vi "FindHome_SingleAxis.vi"(0 "Bd ID In":T3=1, 1 "Home Voltage":dbl, 5 "Axis":T1=1 items=["Axis 1"=1, "Axis 2"=2, "Axis 3"=3, "Axis 4"=4, "Axis 5"=5, "Axis 6"=6, "Axis 7"=7, "Axis 8"=8], 11 "error in":errorcluster, 12 "Velocity (RPM)":i32=65, 13 "Acceleration (RPS/s)":dbl=4.0 format="%.2f") -> (4 "Bd ID Out":T3, 6 "Axis Resource Output":T2 items=["Axis Control"=0, "Axis 1"=1, "Axis 2"=2, "Axis 3"=3, "Axis 4"=4, "Axis 5"=5, "Axis 6"=6, "Axis 7"=7, "Axis 8"=8, "Vector Space Control"=16, "Vector Space 1"=17, "Vector Space 2"=18, "Vector Space 3"=19, "Vector Space 4"=20, "Encoder Control"=32, "Encoder 1"=33, "Encoder 2"=34, "Encoder 3"=35, "Encoder 4"=36, "Encoder 5"=37, "Encoder 6"=38, "Encoder 7"=39, "Encoder 8"=40, "DAC Channel 1"=49, "DAC Channel 2"=50, "DAC Channel 3"=51, "DAC Channel 4"=52, "DAC Channel 5"=53, "DAC Channel 6"=54, "DAC Channel 7"=55, "DAC Channel 8"=56, "Stepper Output 1"=65, "Stepper Output 2"=66, "Stepper Output 3"=67, "Stepper Output 4"=68, "Stepper Output 5"=69, "Stepper Output 6"=70, "Stepper Output 7"=71, "Stepper Output 8"=72, "ADC Channel 1"=81, "ADC Channel 2"=82, "ADC Channel 3"=83, "ADC Channel 4"=84, "ADC Channel 5"=85, "ADC Channel 6"=86, "ADC Channel 7"=87, "ADC Channel 8"=88], 15 "error out":errorcluster)   [LabVIEW 2010]
doc: "Finds home position based on passed in analog voltage value to the closest mill volt and resets encoder counts to zero when found.\n\nNotes:\n\" Although Find Reference VIs are provided by the FlexMotion library, none of them allow for setting an analog voltage value as a reference position. That is what this VI is written for.\n\" Sometimes an axis will not stop at its home position. This is a tuning problem; if the axis is tuned poorly it is unable to stop exactly at the home position."
uses:
  <vilib>/Motion/FlexMotion/CustomControls/CustomControls.llb/Resource Out (Enum).flx
  <vilib>/Motion/FlexMotion/CustomControls/CustomControls.llb/Axis To Control.flx
  <vilib>/Motion/FlexMotion/FunctionsVIs/StartStopMotion.llb/Start Motion (8 axes).flx
  <vilib>/Motion/FlexMotion/FunctionsVIs/Trajectory.llb/Load Accel/Decel in RPS/sec.flx
  <vilib>/Motion/FlexMotion/FunctionsVIs/StartStopMotion.llb/Stop Motion (8 axes).flx
panel:
  out "Pot Voltage":dbl format="%#_4f"
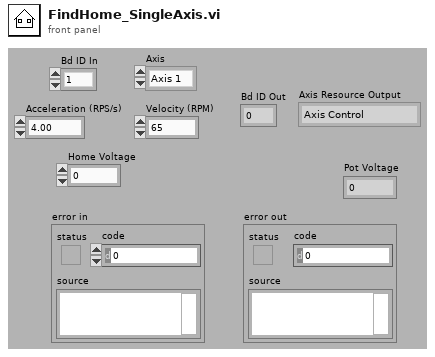
[diagram p1: front panel]
types:
  T1 = typedef "Axis To Control.flx" = u16
  T2 = typedef "Resource Out (Enum).flx" = u16
  T3 = typedef "Bd Id Out" = u8
  T4 = enum16{"Absolute Position", "Relative Position", "Velocity", "Relative to Cap Pos", "Modulus Position", "Absolute Contouring", "Relative Contouring"}
  T5 = cluster{"Run/Stop":bool, "Profile Complete":bool, "Motor Off ":bool, "Following Error":bool, "Limit Switch":bool, "Home Switch":bool, "SW Limit Switch":bool, "Watchdog":bool, "Velocity Threshold":bool, "Position Brkpt":bool, "Home Found":bool, "Index Found":bool, "High Speed Capture":bool, "Reverse Direction":bool, "Blend Complete":bool, "Move Complete":bool}
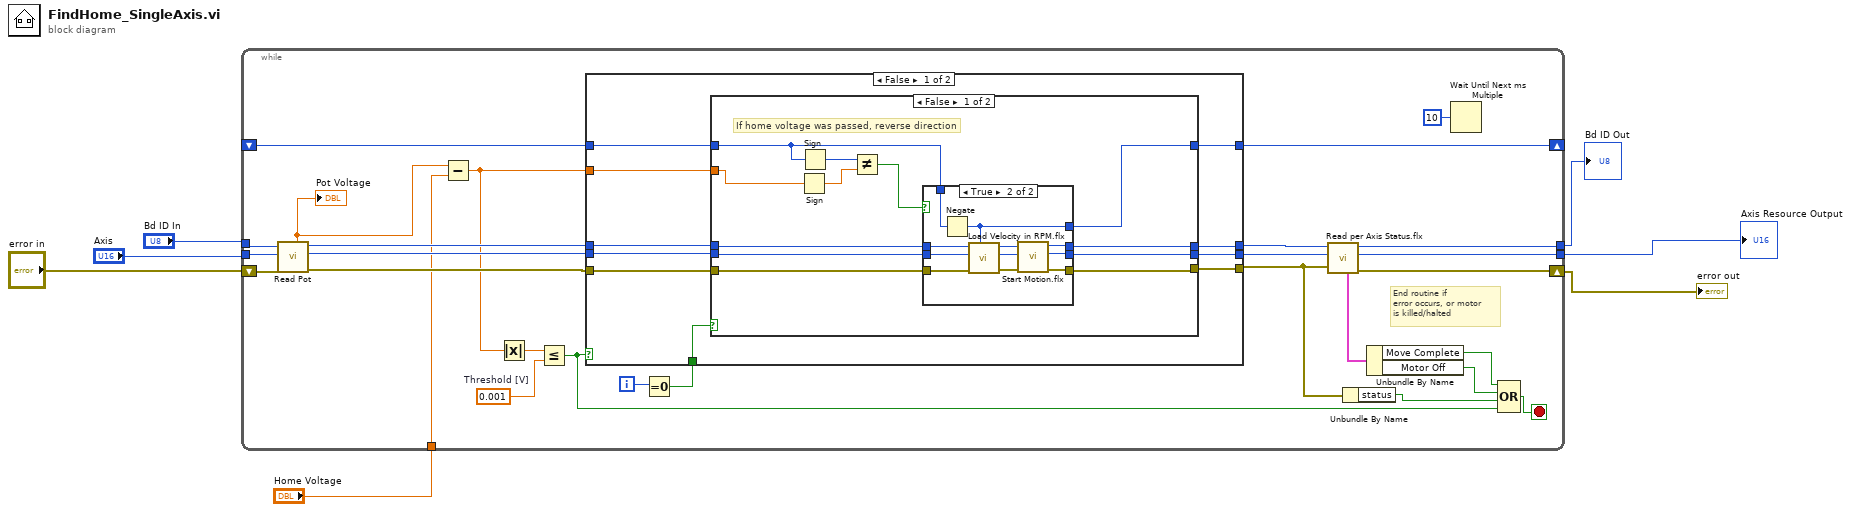
[diagram p0: block diagram]
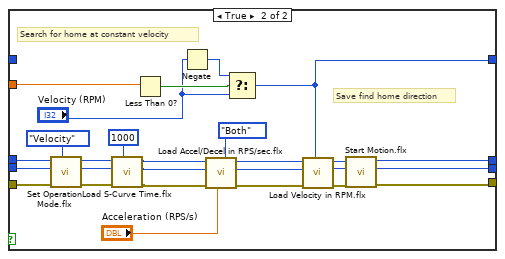
[diagram p3: hidden frame]
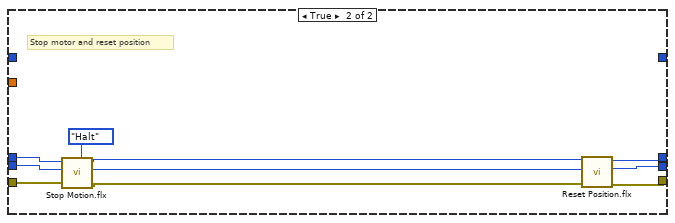
[diagram p4: hidden frame]
diagram:
  n1 = while {
    tunnel: "Bd ID In" -> [w29]
    tunnel: [w19] -> w7
    tunnel: [w18] -> w6
    shift-right: [w21] -> w5
    shift-left: "error in" -> [w26]
    tunnel: "Axis" -> [w15]
    tunnel: "Home Voltage" -> [w12]
    shift-right: [w10] -> _
    shift-left: _ -> [w9]
    i -> [w34]
    stop <- w33 stop-if-true
    w35 = 0.001  # Threshold [V]
    # "End routine if\nerror occurs, or motor\nis killed/halted"
    n2 = call "Read Pot.vi"("error in (no error)"=w26, "Axis In"=w15, "Board ID"=w29) -> ("error out"=w25:errorcluster, "Axis Out"=w27:T1, "Bd ID Out"=w28:T3, "Pot Voltage"=w14:dbl)  [unwired: 5 in]
    "Pot Voltage" <- w14
    n3 = Subtract(x=w14, y=w12) -> (x-y=w24:dbl)
    n4 = Absolute Value(x=w24) -> (abs(x)=w32:dbl)
    n5 = Less Or Equal?(x=w32, y=w35) -> (x <= y?=w8:bool)
    n6 = Equal To 0?(x=w34) -> (x = 0?=w30:bool)
    n7 = case shown="False" w8 {
      tunnel: [w45 w108] -> w23
      tunnel: [w44 w107] -> w22
      tunnel: [w43 w106] -> w20
      tunnel: w28 -> [w41 w105]
      tunnel: w30 -> [w42 _]
      tunnel: w24 -> [w40 _]
      tunnel: w27 -> [w39 w101]
      tunnel: w25 -> [w38 w100]
      tunnel: [w37 _] -> w10
      tunnel: w9 -> [w36 _]
      frame False {
        n8 = case shown="False" w42 {
          tunnel: [w53 w99] -> w45
          tunnel: [w54 w98] -> w44
          tunnel: [w56 w97] -> w43
          tunnel: w41 -> [w51 w89]
          tunnel: w40 -> [w52 w93]
          tunnel: w39 -> [w50 w88]
          tunnel: w38 -> [w49 w90]
          tunnel: [w46 w74] -> w37
          tunnel: w36 -> [w47 _]
          frame False {
            # "If home voltage was passed, reverse direction"
            n9 = Sign(1:w52) -> (0:w57:dbl)
            n10 = Sign(1:w47) -> (0:w48:i32)
            n11 = Not Equal?(x=w48, y=w57) -> (x != y?=w55:bool)
            n12 = case shown="True" w55 {
              tunnel: [w59 w66] -> w56
              tunnel: w49 -> [w59 w72]
              tunnel: w51 -> [w61 w70]
              tunnel: w50 -> [w60 w71]
              tunnel: [w61 w62] -> w53
              tunnel: [w60 w65] -> w54
              tunnel: w47 -> [w58 w69]
              tunnel: [w58 w68] -> w46
              frame False {
              }
              frame True {
                n13 = Negate(x=w69) -> (-x=w68:i32)
                n14 = call <vilib>:"Load Velocity in RPM.flx"("Velocity (500)"=w68, "error in (no error)"=w72, "Axis or Vector Space"=w71, "Board ID"=w70) -> ("error out"=w67:errorcluster, "Resource Output"=w64:T2, "Bd ID Out"=w63:T3)  [unwired: 3 in]
                n15 = call-poly <vilib>:"Start Motion.flx"("error in (no error)"=w67, "Axis or Vector Space"=w64, "Board ID"=w63) -> ("error out"=w66:errorcluster, "Resource Output"=w65:T2, "Bd ID Out"=w62:T3)  [unwired: 3 in]
              }
            }
          }
          frame True {
            # "Save find home direction"
            # "Search for home at constant velocity"
            n16 = call <vilib>:"Set Operation Mode.flx"("Position Mode (Absolute)"=T4."Velocity", "error in (no error)"=w90, "Axis or Vector Space"=w88, "Board ID"=w89) -> ("error out"=w86:errorcluster, "Resource Output"=w84:T2, "Bd ID Out"=w85:T3)  [unwired: 2 in]
            n17 = call <vilib>:"Load S-Curve Time.flx"("S Curve Time (1)"=u16 1000, "error in (no error)"=w86, "Axis or Vector Space"=w84, "Board ID"=w85) -> ("error out"=w80:errorcluster, "Resource Output"=w81:T2, "Bd ID Out"=w82:T3)  [unwired: 3 in]
            n18 = Less Than 0?(x=w93) -> (x < 0?=w79:bool)
            n19 = Negate(x="Velocity (RPM)") -> (-x=w78:i32)
            n20 = call "Load Accel/Decel in RPS/sec.flx"("Selector (Both)"=enum16{"Both", "Acceleration", "Deceleration"}."Both" ("Acceleration Type (Both)"), "Value (200)"="Acceleration (RPS/s)", "error in (no error)"=w80, "Axis or Vector Space"=w81, "Board ID"=w82) -> ("error out"=w75:errorcluster, "Resource Output"=w76:T2, "Bd ID Out"=w77:T3)  [unwired: 2 in]
            n21 = Select(t=w78, s=w79, f="Velocity (RPM)") -> (s? t:f=w74:i32)
            n22 = call <vilib>:"Load Velocity in RPM.flx"("Velocity (500)"=w74, "error in (no error)"=w75, "Axis or Vector Space"=w76, "Board ID"=w77) -> ("error out"=w96:errorcluster, "Resource Output"=w95:T2, "Bd ID Out"=w94:T3)  [unwired: 3 in]
            n23 = call-poly <vilib>:"Start Motion.flx"("error in (no error)"=w96, "Axis or Vector Space"=w95, "Board ID"=w94) -> ("error out"=w97:errorcluster, "Resource Output"=w98:T2, "Bd ID Out"=w99:T3)  [unwired: 3 in]
          }
        }
      }
      frame True {
        # "Stop motor and reset position"
        n24 = call-poly <vilib>:"Stop Motion.flx"("Stop Type (Decel)"=enum16{"Decelerate", "Halt", "Kill"}."Halt", "error in (no error)"=w100, "Axis or Vector Space"=w101, "Board ID"=w105) -> ("error out"=w102:errorcluster, "Resource Output"=w103:T2, "Bd ID Out"=w104:T3)  [unwired: 3 in]
        n25 = call <vilib>:"Reset Position.flx"("error in (no error)"=w102, "Axis"=w103, "Board ID"=w104) -> ("error out"=w106:errorcluster, "Resource Output"=w107:T2, "Bd ID Out"=w108:T3)  [unwired: 4 in]
      }
    }
    n26 = call <vilib>:"Read per Axis Status.flx"("error in (no error)"=w20, "Axis"=w22, "Board ID"=w23) -> ("error out"=w21:errorcluster, "Resource Output"=w18:T2, "Bd ID Out"=w19:T3, "Per Axis H/W Status"=w17:T5)  [unwired: 3 in]
    n27 = Unbundle By Name(w20) -> ("status"=w31:bool)
    n28 = Unbundle By Name(w17) -> ("Move Complete"=w13:bool, "Motor Off"=w16:bool)
    n29 = Wait Until Next ms Multiple(millisecond multiple=u32 10) -> ()  [unwired: 1 out]
    n30 = Compound Arithmetic op=OR(w13, w16, w31, w8) -> (w33:bool)
  }
  "Bd ID Out" <- w7
  "error out" <- w5
  "Axis Resource Output" <- w6
